vi "OpenXL_WorkSheet By Name.vi"(8 "error in (no error)":errorcluster, 10 "SheetName(\"\")":string, 11 "Refnum Cluster In":T1) -> (0 "error out":errorcluster, 3 "Refnum Cluster Out":T2)   [LabVIEW 2015]
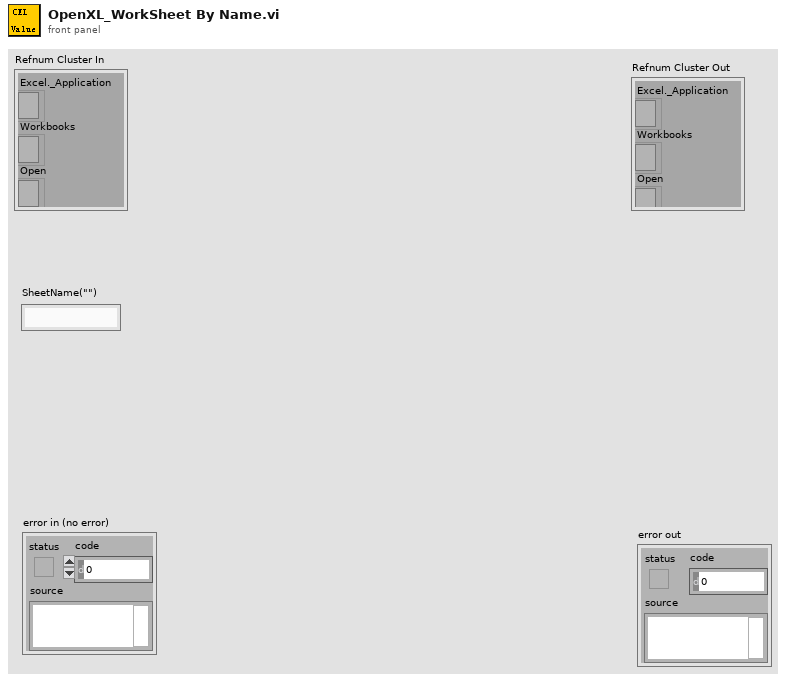
[diagram p1: front panel]
types:
  T1 = cluster{"Excel._Application":refnum<k7>, "Workbooks":refnum<k7>, "Open":refnum<k7>}
  T2 = cluster{"Excel._Application":refnum<k7>, "Workbooks":refnum<k7>, "Open":refnum<k7>, "Worksheets":refnum<k7>, "Excel._Worksheet":refnum<k7>}
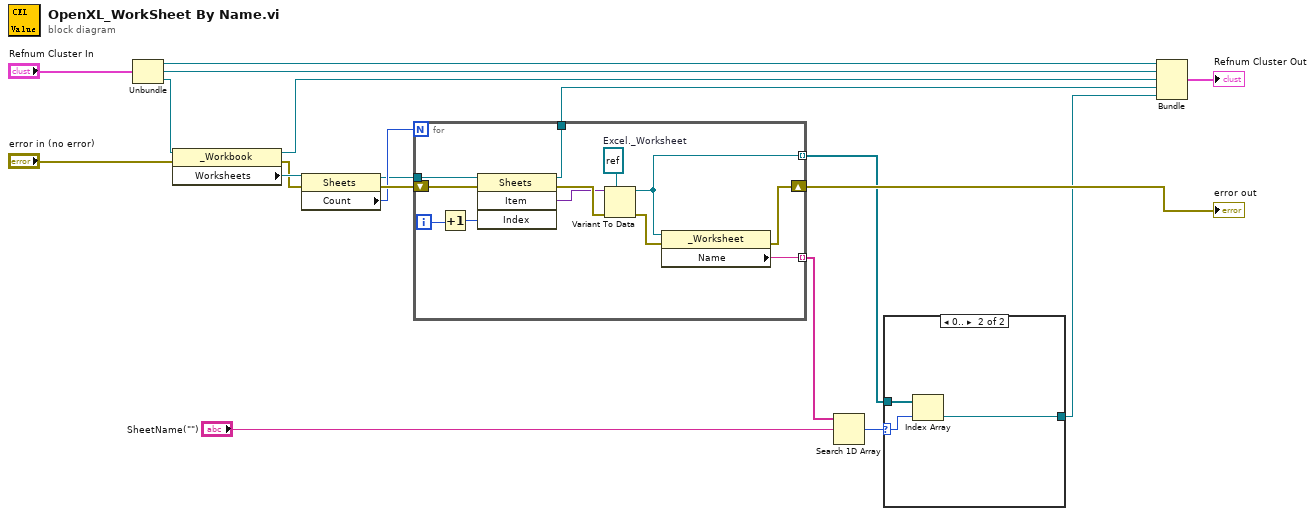
[diagram p0: block diagram]
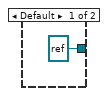
[diagram p2: hidden frame]
diagram:
  n1 = Unbundle("Refnum Cluster In") -> ("Excel._Application"=w15:refnum<k7>, "Workbooks"=w16:refnum<k7>, "Open"=w14:refnum<k7>)
  n2 = property class="_Workbook"(reference=w14, error in="error in (no error)") -> (reference out=w18:refnum<k7>, error out=w9:errorcluster, "Worksheets"=w10:refnum<k7>)
  n3 = property class="Sheets"(reference=w10, error in=w9) -> (reference out=w1:refnum<k7>, error out=w8:errorcluster, "Count"=w7:i32)
  n4 = for {
    N: w7 -> [_]
    tunnel: [w31] -> w19
    shift-right: [w25] -> w17
    shift-left: w8 -> [w27]
    tunnel: [w24] -> w3 mode=indexing
    tunnel: [w23] -> w6 mode=indexing
    tunnel: w1 -> [w22]
    i -> [w21]
    w29 = refnum<k7> refnum  # Excel._Worksheet
    n5 = Increment(x=w21) -> (x+1=w20:i32)
    n6 = invoke class="Sheets" method="Item"(reference=w22, error in=w27, "Index"=w20) -> (reference out=w31:refnum<k7>, error out=w30:errorcluster, "Item"=w28:variant)  [unwired: 1 in, 1 out]
    n7 = Variant To Data(error in=w30, type=w29, Variant=w28) -> (data=w24:refnum<k7>, error out=w26:errorcluster)
    n8 = property class="_Worksheet"(reference=w24, error in=w26) -> (error out=w25:errorcluster, "Name"=w23:string)  [unwired: 1 out]
  }
  "error out" <- w17
  n9 = Search 1D Array(1D array=w6, element="SheetName(\"\")") -> (index of element=w4:i32)  [unwired: 1 in]
  n10 = case shown="0.." w4 {
    selector: w4 -> [_ w34]
    tunnel: w3 -> [_ w35]
    tunnel: [refnum<k7> refnum ("Excel._Worksheet") w33] -> w2
    frame Default {
    }
    frame 0.. {
      n11 = Index Array(array=w35, index=w34) -> (element=w33:refnum<k7>)
    }
  }
  n12 = Bundle("Excel._Application"=w15, "Workbooks"=w16, "Open"=w18, "Worksheets"=w19, "Excel._Worksheet"=w2) -> (→"Refnum Cluster Out":T2)  [unwired: 1 in]
